vi "Read Register.vi"   [LabVIEW 2020, in "SLSC.lvlib"]
doc: "Reads from the given <B>register address</B> of the specified <B>device</B>."
uses:
  <vilib>/SLSC/SLSC.lvlib
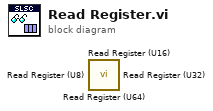
[diagram p0: block diagram]
diagram:
  n1 = call <vilib>:"Read Register (U64).vi"() -> ()  [unwired: 11 in, 5 out]
  n2 = call <vilib>:"Read Register (U16).vi"() -> ()  [unwired: 11 in, 5 out]
  n3 = call <vilib>:"Read Register (U8).vi"() -> ()  [unwired: 11 in, 5 out]
  n4 = call <vilib>:"Read Register (U32).vi"() -> ()  [unwired: 11 in, 5 out]
